vi "Check Stream OK.vi"(8 "error in (no error)":errorcluster, 11 "Camera in":refnum<class "Camera.lvclass">) -> (0 "error out":errorcluster)   [LabVIEW 2020, in "Camera.lvclass"]
uses:
  Camera.lvclass
  Camera.lvclass/Camera.ctl
  <vilib>/Utility/error.llb/Error Cluster From Error Code.vi
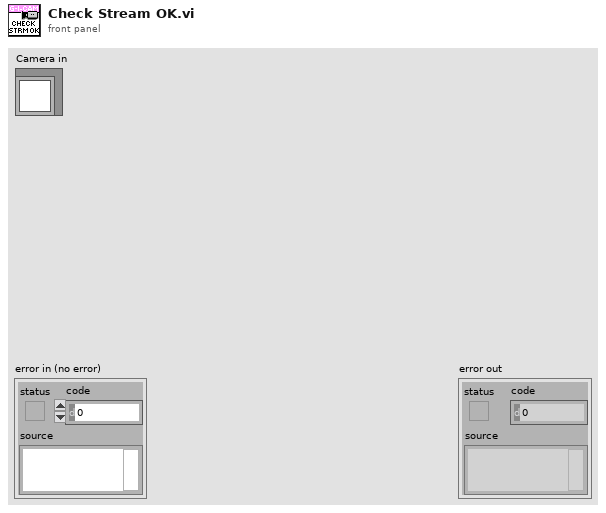
[diagram p1: front panel]
types:
  T1 = typedef "Camera.lvclass/Streaming Registation.ctl" = cluster{"Streaming Events":refnum<event-registration>, "User Events":T2}
  T2 = typedef "Camera.lvclass/Stream User Events.ctl" = cluster{"Stopped":refnum<user-event>, "Errors":refnum<user-event>}
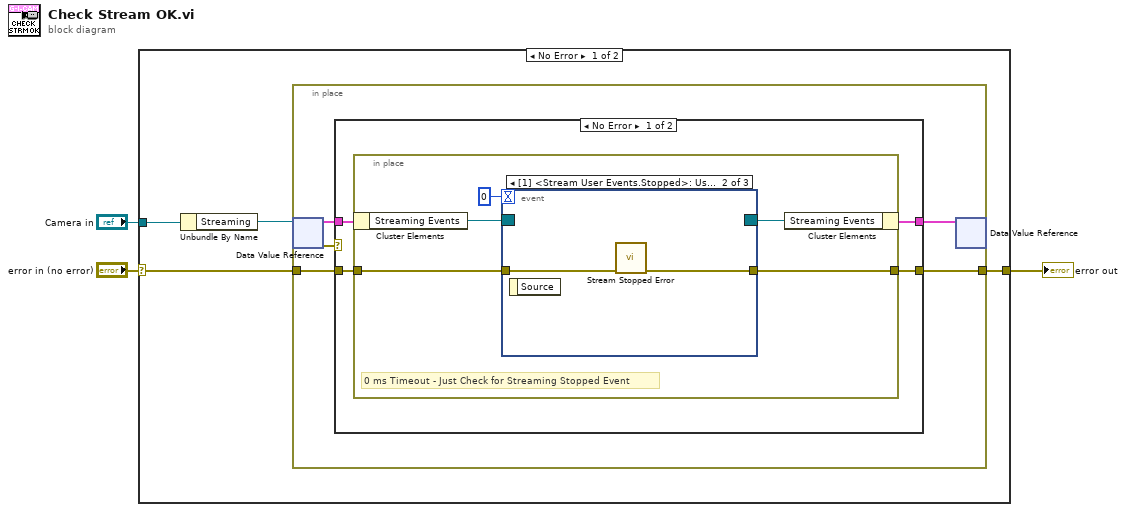
[diagram p0: block diagram]
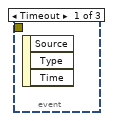
[diagram p2: hidden frame]
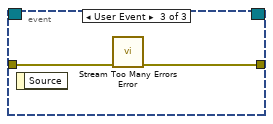
[diagram p3: hidden frame]
diagram:
  n1 = case shown="No Error" "error in (no error)" {
    selector: "error in (no error)" -> [w5 w28]
    tunnel: [w4 w28] -> w2
    tunnel: "Camera in" -> [w7 _]
    frame No Error {
      n2 = Unbundle By Name(w7) -> ("Streaming"=w6:refnum<data-value>)
      n3 = in-place {
        in-place-border: w5 -> [w9]
        in-place-border: [w8] -> w4
        n4 = in-place-dvr #1(w6) -> (w11:T1, w12:errorcluster)
        n5 = case shown="No Error" w12 {
          selector: w12 -> [_ w26]
          tunnel: w11 -> [w16 w27]
          tunnel: [w15 w27] -> w10
          tunnel: w9 -> [w14 _]
          tunnel: [w13 w26] -> w8
          frame No Error {
            n6 = in-place {
              in-place-border: w14 -> [w18]
              in-place-border: [w17] -> w13
              # "0 ms Timeout - Just Check for Streaming Stopped Event"
              n7 = in-place-cluster #2(w16) -> ("Streaming Events"=w20:refnum<event-registration>)
              n8 = event shown="[1] <Stream User Events.Stopped>: User Event" {
                selector: w20 -> [_ _ _]
                dyn-events: [_ _ _] -> w19
                timeout: 0 -> [_ _ _]
                tunnel: w18 -> [_ w23 w25]
                tunnel: [_ w22 w24] -> w17
                event Timeout {
                  n9 = event-data() -> ()  [unwired: 1 in, 3 out]
                }
                event User Event {
                  n10 = event-data() -> ()  [unwired: 1 in, 1 out]
                  n11 = call "Stream Stopped Error.vi"("error in (no error)"=w23) -> ("error out"=w22:errorcluster)  [unwired: 10 in]
                }
                event User Event {
                  n12 = event-data() -> ()  [unwired: 1 in, 1 out]
                  n13 = call "Stream Too Many Errors Error.vi"("error in (no error)"=w25) -> ("error out"=w24:errorcluster)  [unwired: 10 in]
                }
              }
              n14 = in-place-cluster #2("Streaming Events"=w19) -> (w15:T1)
            }
          }
          frame Error {
          }
        }
        n15 = in-place-dvr #1(w10) -> ()  [unwired: 2 out]
      }
    }
    frame Error {
    }
  }
  "error out" <- w2
